vi "禹山叶绿素a校准.vi"() -> ()   [LabVIEW 2016, in "斯坦道多参数.lvlib"]
uses:
  <vilib>/Utility/miscctls.llb/LVPointTypeDef.ctl
  <vilib>/Analysis/NI_AALBase.lvlib
  <vilib>/Analysis/NI_AALPro.lvlib
  <vilib>/Utility/config.llb/NI_LVConfig.lvlib
panel:
  out "第二点校准值":dbl
  out "第一点校准值":dbl
  out "最小值":sgl format="%.2g"
  out "最大值":sgl format="%.2g"
  in  "校准停止":bool
  in  "校准模式":enum16{"两点校准", "单点校准"}(ring)
  in  "标液2":dbl
  in  "标液1":dbl
  out "波形图表":sgl(graph) caption="历史曲线"
  out "温度测量值":dbl caption="温度"
  out "变异系数":dbl format="%.6g"
  out "standard deviation":dbl caption="标准差" format="%0.2f"
  out "mean":dbl caption="均值" format="%0.2f"
  out "提示":string
  in  "校准启动":bool
  out "测试值":dbl
  out "电极斜率":dbl
  out "电极零点":dbl
  # "叶绿素a电极设定"
  # "请选择校准模式:"
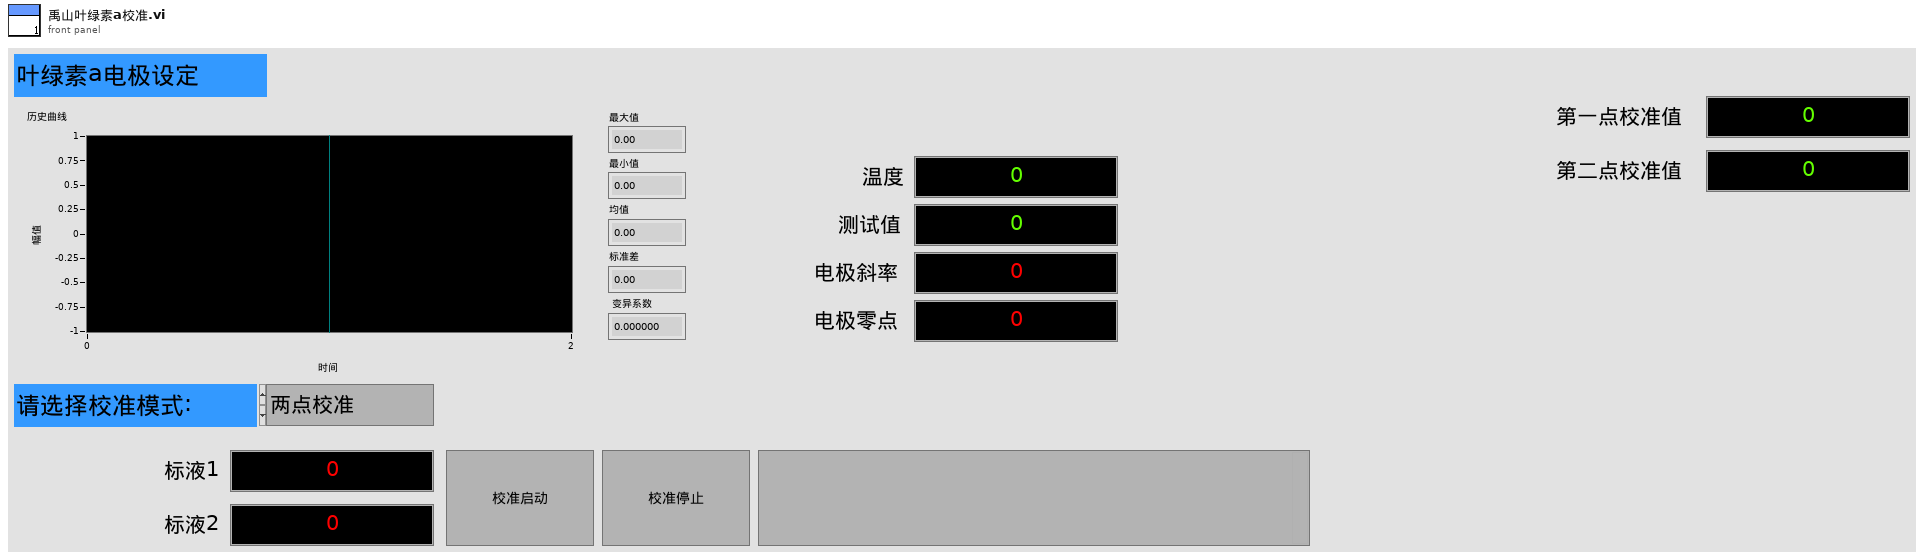
[diagram p1: front panel]
types:
  T1 = typedef "斯坦道多参数.lvlib/校准步骤.ctl" = enum16{"待机", "放置第一点标液", "第一点校准启动", "第一点校准写入", "第一点校准失败", "放置第二点标液", "第二点校准启动", "第二点校准写入", "第二点校准失败", "校准结果写入", "校准结束"}
  T2 = typedef "LVPointTypeDef.ctl" = cluster{"Horizontal":i16, "Vertical":i16}
  T3 = typedef "NI_LVConfig.lvlib/Config Data RefNum.ctl" = refnum<k1>
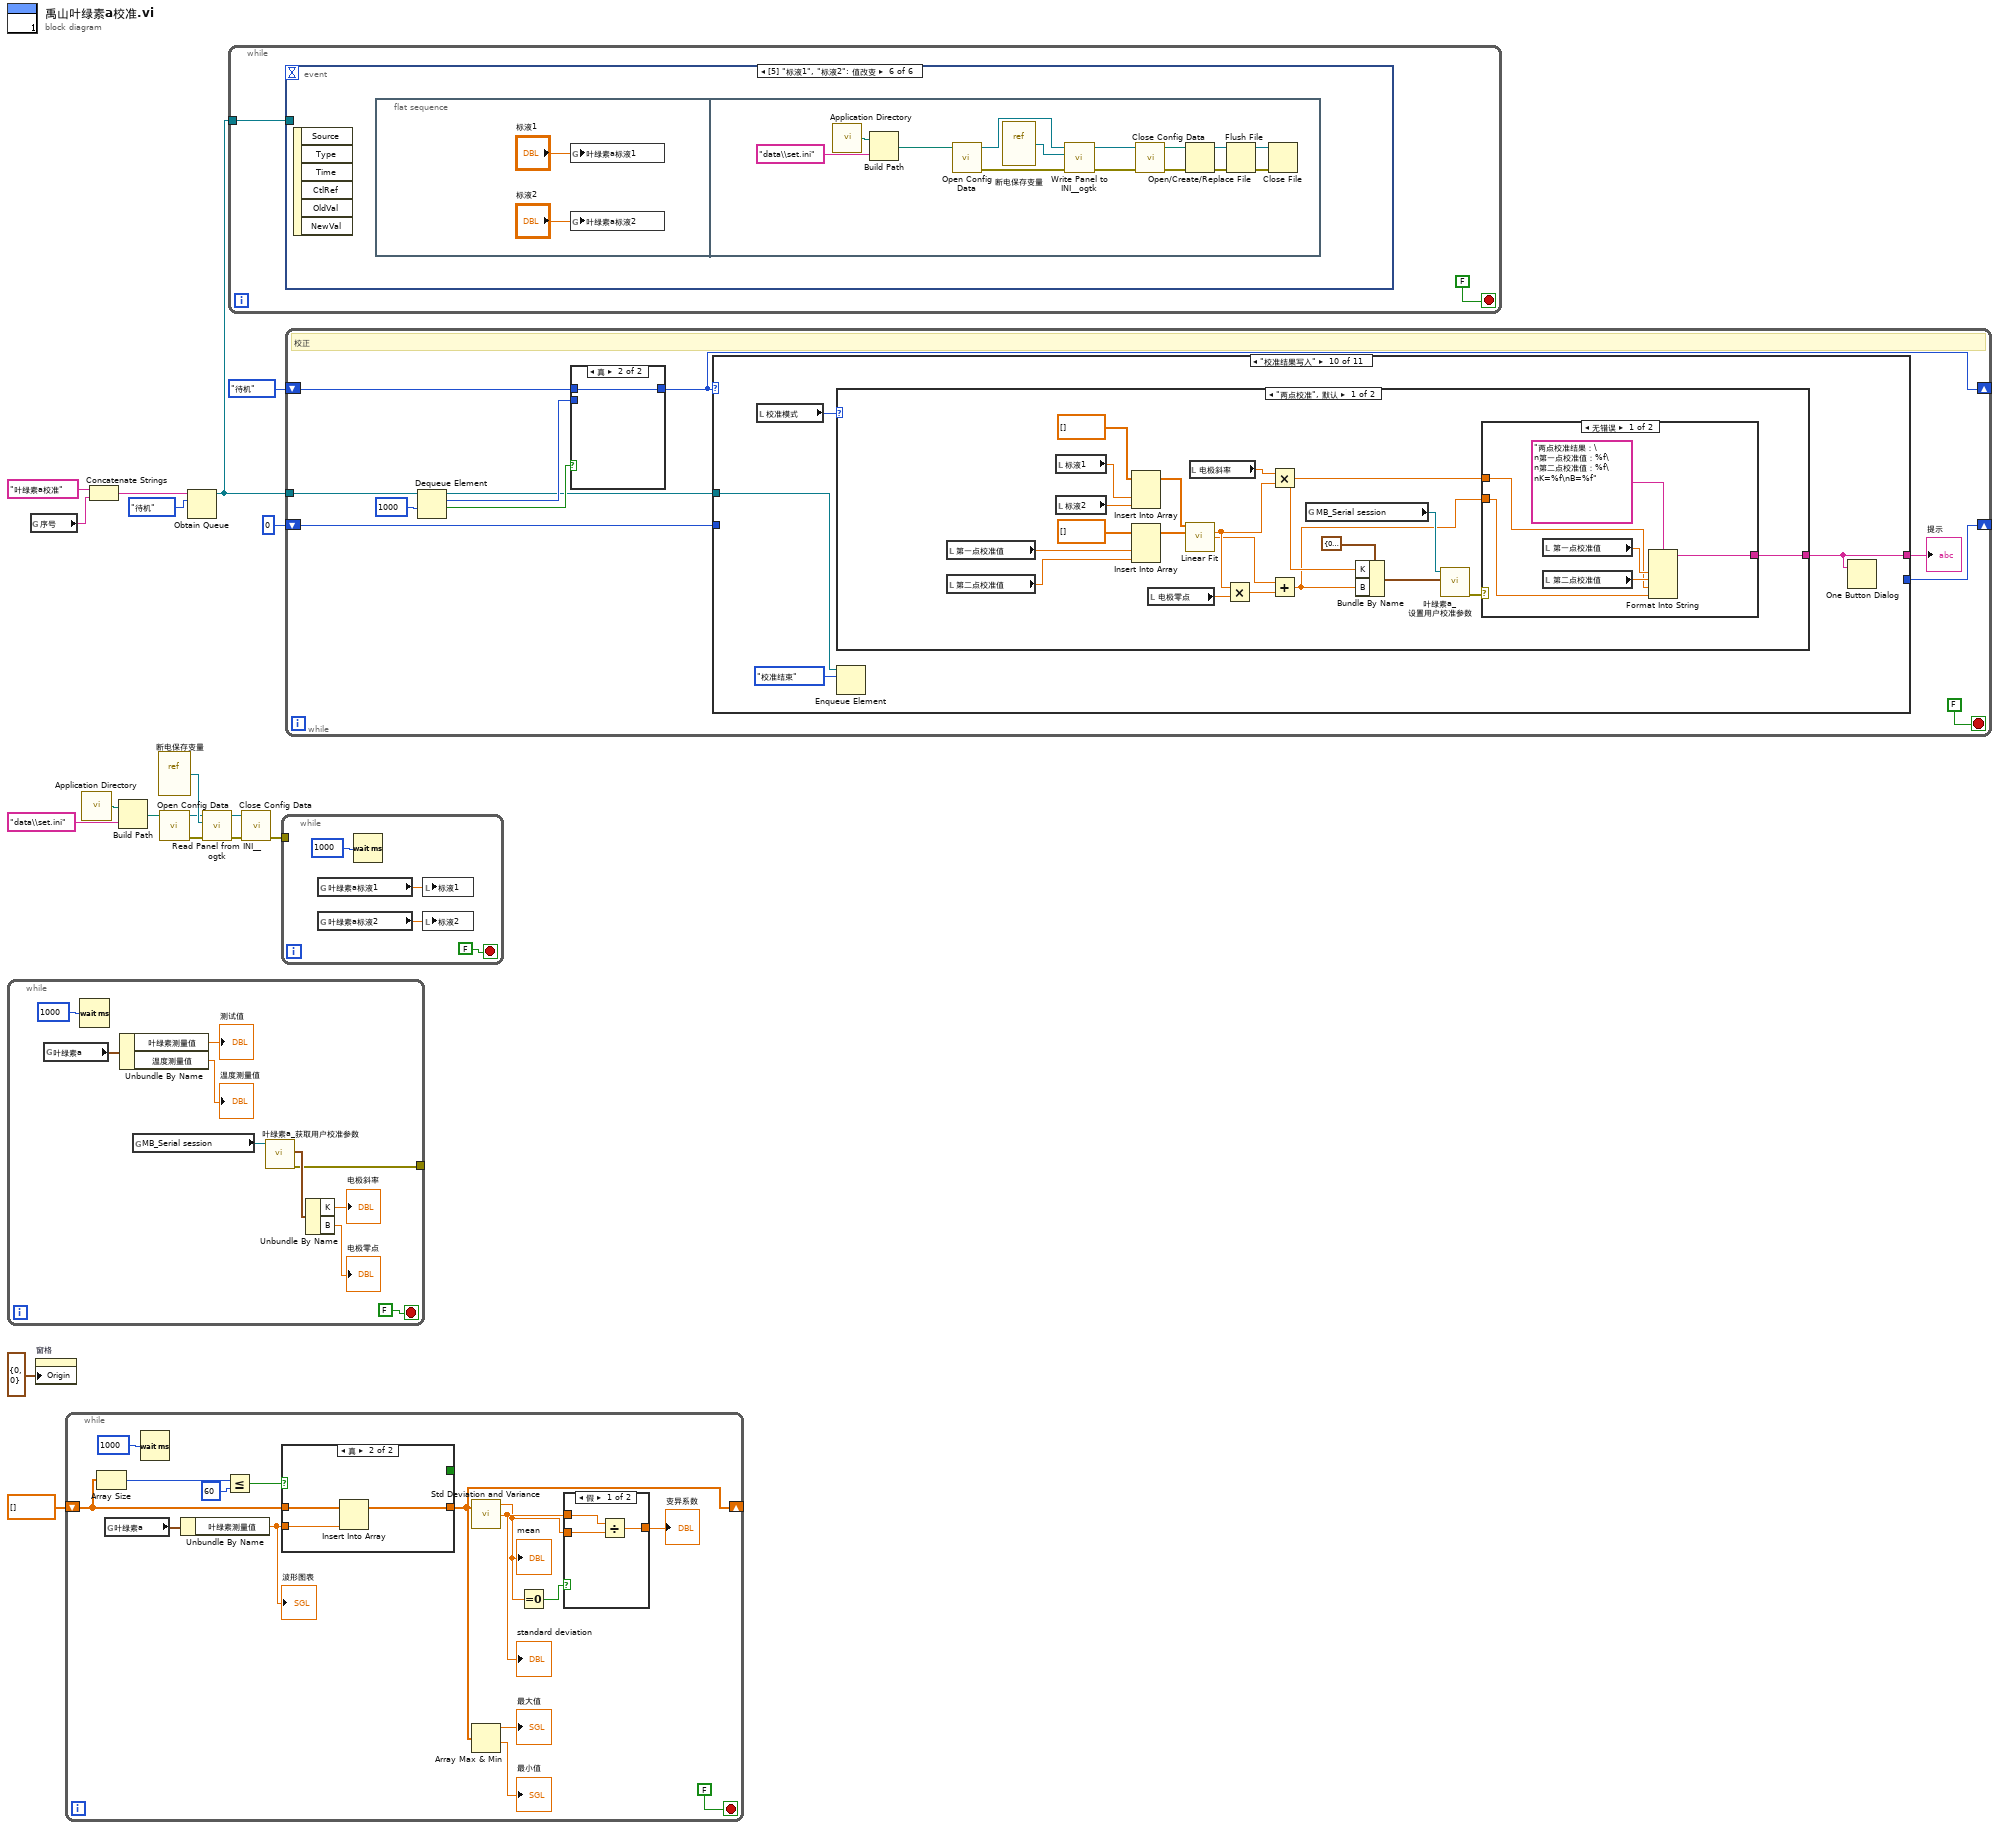
[diagram p0: block diagram]
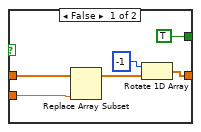
[diagram p3: hidden frame]
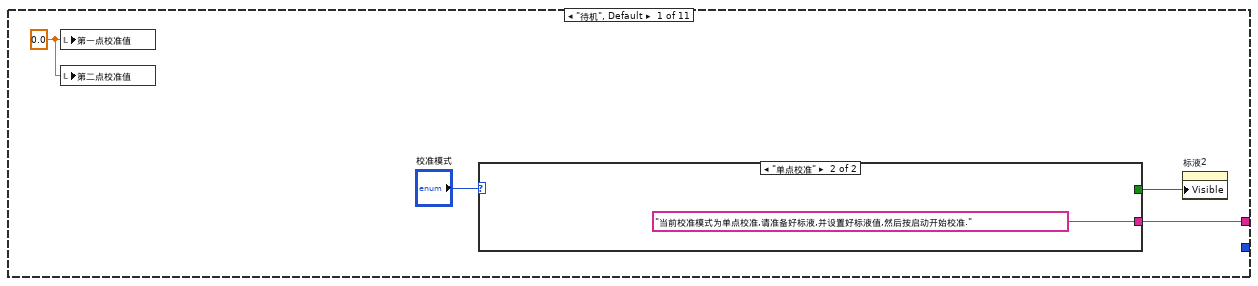
[diagram p5: hidden frame]
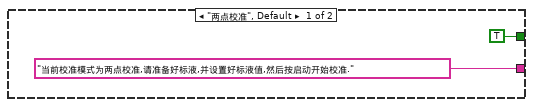
[diagram p6: hidden frame]
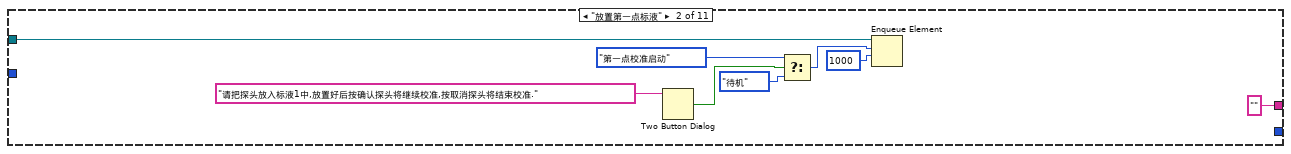
[diagram p7: hidden frame]
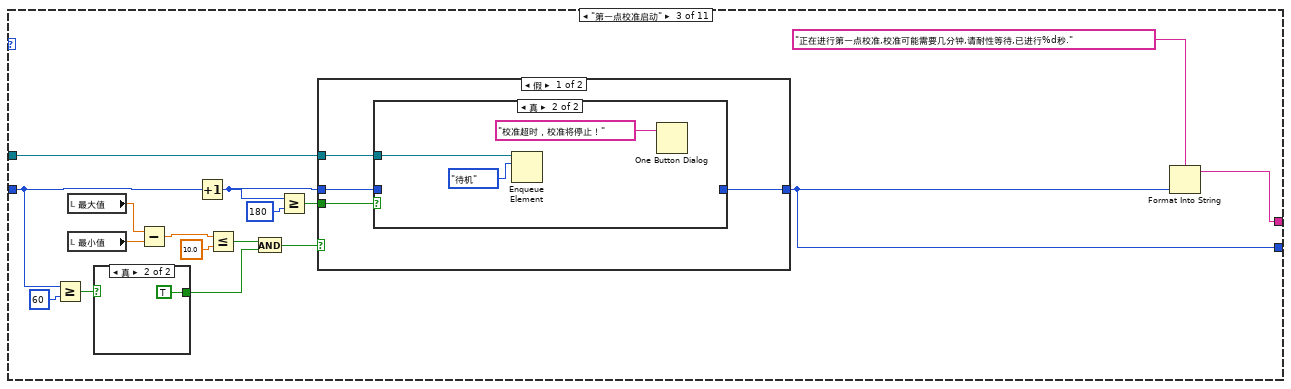
[diagram p8: hidden frame]
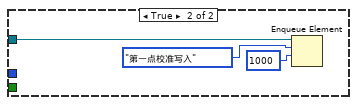
[diagram p10: hidden frame]
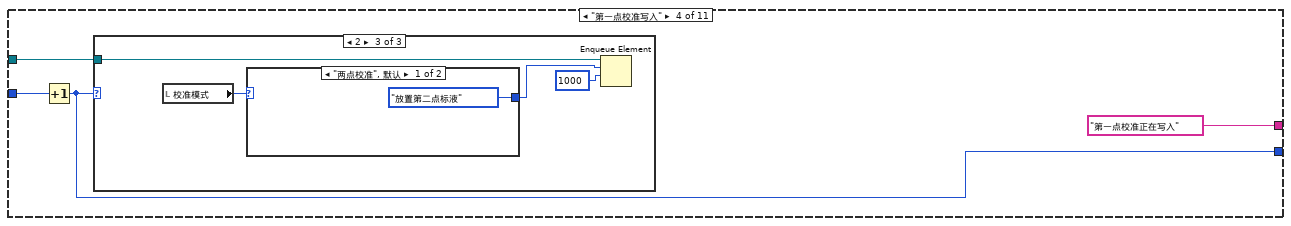
[diagram p12: hidden frame]
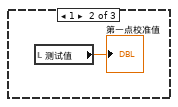
[diagram p14: hidden frame]
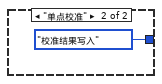
[diagram p15: hidden frame]
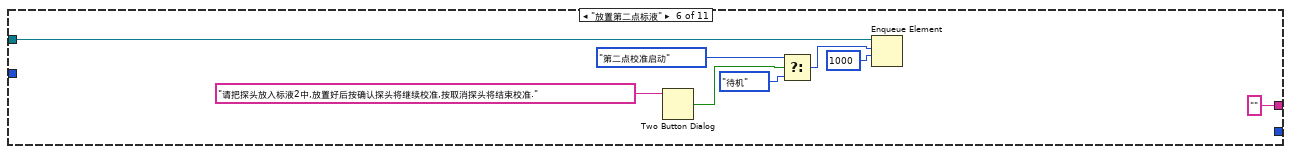
[diagram p17: hidden frame]
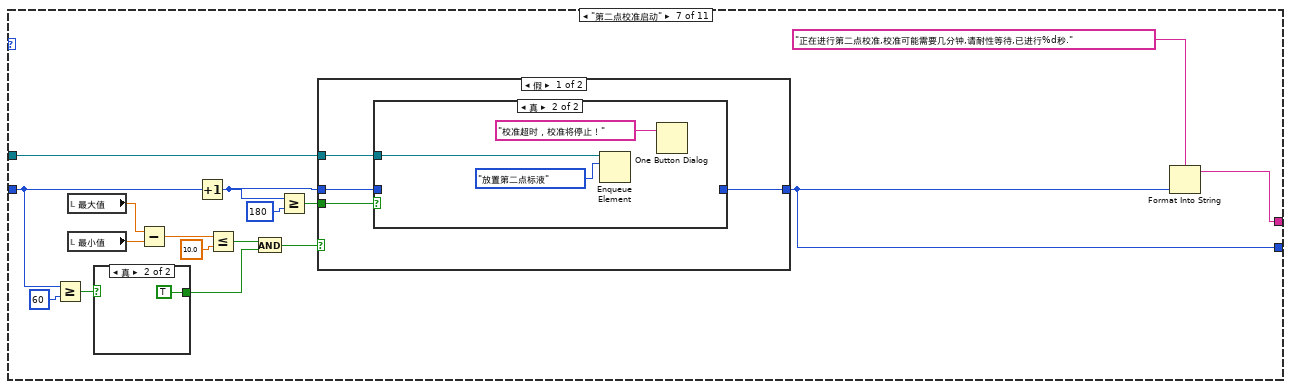
[diagram p18: hidden frame]
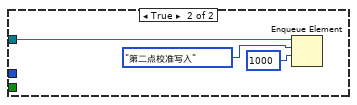
[diagram p20: hidden frame]
diagram:
  n1 = while {
    tunnel: [w23] -> _
    stop <- FALSE stop-if-true
    n2 = global read "禹山过程全局变量.vi" "叶绿素a"() -> (w20:cluster{"温度测量值":sgl, "叶绿素测量值":sgl, "错误标志":u16})
    n3 = Wait (ms)(milliseconds to wait=u32 1000 ("等待时间（毫秒）")) -> ()  [unwired: 1 out]
    n4 = Unbundle By Name(w20) -> ("叶绿素测量值"=→"测试值":sgl, "温度测量值"=→"温度测量值":sgl)
    n5 = global read "多参数全局变量.vi" "MB_Serial session"() -> (w19:refnum<class "MB_Master_Serial.lvclass">)
    n6 = call "叶绿素a_获取用户校准参数.vi"("MB_Serial session in"=w19) -> ("error out"=w23:errorcluster, "输出值"=w26:cluster{"K":sgl, "B":sgl})  [unwired: 8 in, 1 out]
    n7 = Unbundle By Name(w26) -> ("K"=→"电极斜率":sgl, "B"=→"电极零点":sgl)
  }
  n8 = global read "多参数全局变量.vi" "序号"() -> (w1:string)
  n9 = property on="窗格" class="Pane"("Origin"=T2 {"Horizontal"=0, "Vertical"=0} ("原点")) -> ()  [unwired: 2 in, 2 out]
  n10 = while {
    shift-right: [w31] -> _
    shift-left: sgl[] [] -> [w39]
    stop <- FALSE stop-if-true
    n11 = Array Size(array=w39) -> (size(s)=w41:i32)
    n12 = global read "禹山过程全局变量.vi" "叶绿素a"() -> (w33:cluster{"温度测量值":sgl, "叶绿素测量值":sgl, "错误标志":u16})
    n13 = Wait (ms)(milliseconds to wait=u32 1000 ("等待时间（毫秒）")) -> ()  [unwired: 1 out]
    n14 = Unbundle By Name(w33) -> ("叶绿素测量值"=w32:sgl)
    "波形图表" <- w32
    n15 = Less Or Equal?(x=w41, y=60) -> (x <= y?=w40:bool)
    n16 = case shown="真" w40 {
      tunnel: w39 -> [w52 w55]
      tunnel: w32 -> [w50 w54]
      tunnel: [w48 w53] -> w31
      tunnel: [TRUE _] -> _
      frame False {
        n17 = Replace Array Subset(array=w52, new element=w50) -> (w51:sgl[])  [unwired: 1 in]
        n18 = Rotate 1D Array(1:w51, 2:-1 ("n")) -> (0:w48:sgl[])
      }
      frame True {
        n19 = Insert Into Array(array=w55, new element=w54) -> (w53:sgl[])  [unwired: 1 in]
      }
    }
    n20 = call <vilib>:"Std Deviation and Variance.vi"("X"=w31) -> ("mean"=w34:dbl, "standard deviation"=w35:dbl)  [unwired: 1 in, 1 out]
    "standard deviation" <- w35
    "mean" <- w34
    n21 = Array Max & Min(array=w31) -> (max value=→"最大值":sgl, min value=→"最小值":sgl)  [unwired: 2 out]
    n22 = Equal To 0?(x=w34) -> (x = 0?=w38:bool)
    n23 = case shown="假" w38 {
      tunnel: w35 -> [w46 _]
      tunnel: [w45 _] -> w37
      tunnel: w34 -> [w44 _]
      frame False {
        n24 = Divide(x=w46, y=w44) -> (x/y=w45:dbl)
      }
      frame True {
      }
    }
    "变异系数" <- w37
  }
  n25 = call <vilib>:"Application Directory.vi"() -> ("Application Directory"=w8:path)
  n26 = Concatenate Strings("叶绿素a校准" ("名称（未命名）"), w1) -> (w2:string)
  n27 = Build Path(base path=w8, name or relative path="data\\set.ini" ("名称或相对路径")) -> (appended path=w9:path)
  n28 = vi-ref "断电保存变量.vi"() -> (w11:refnum<vi>)
  n29 = call <vilib>:"Open Config Data.vi"("configuration file path"=w9) -> ("error out"=w5:errorcluster, "refnum"=w4:T3)  [unwired: 8 in, 1 out]
  n30 = Obtain Queue(name (unnamed)=w2, element data type=校准步骤."待机" ("枚举")) -> (queue out=w12:refnum<queue>)  [unwired: 3 in, 2 out]
  n31 = call <userlib>:"Read Panel from INI__ogtk.vi"("error in (no error)"=w5, "VI ref"=w11, "refnum"=w4) -> ("error out"=w7:errorcluster, "refnum out"=w6:T3)  [unwired: 7 in]
  n32 = while {
    tunnel: w12 -> [w56]
    stop <- FALSE stop-if-true
    n33 = event shown="[5] \"标液1\", \"标液2\": 值改变" {
      selector: _ -> [_ _ _ _ _ _]
      dyn-events: _ -> [_ _ _ _ _ _]
      timeout: _ -> [_ _ _ _ _ _]
      tunnel: w56 -> [_ w59 w63 _ _ _]
      event Timeout {
        n34 = event-data() -> ()  [unwired: 1 in, 3 out]
      }
      event "校准启动": Value Change {
        n35 = event-data() -> ()  [unwired: 1 in, 6 out]
        n36 = Enqueue Element(queue=w59, element=校准步骤."放置第一点标液" ("元素")) -> ()  [unwired: 2 in, 3 out]
      }
      event "校准停止": Value Change {
        n37 = event-data() -> ()  [unwired: 1 in, 6 out]
        n38 = Flush Queue(queue=w63) -> (queue out=w60:refnum<queue>)  [unwired: 1 in, 2 out]
        n39 = Enqueue Element(queue=w60, element=校准步骤."待机" ("元素"), timeout in ms (-1)=1000 ("超时毫秒(-1)")) -> ()  [unwired: 1 in, 3 out]
      }
      event "电极零点", "电极斜率", "标液1", "标液2": Mouse Down {
        n40 = event-data() -> ("CtlRef"=w64:refnum<vi>)  [unwired: 1 in, 7 out]
        n41 = property class="DigNum (严格)"(reference=w64) -> (reference out=w65:refnum<vi>, "Value"=w66:dbl)  [unwired: 1 in, 1 out]
        n42 = call "数字键盘.vi"("OldNumber"=w66) -> ("NewNumber"=w67:sgl)
        n43 = property class="DigNum (严格)"(reference=w65, "Val(Sgnl)"=w67) -> ()  [unwired: 1 in, 2 out]
      }
      event "电极零点", "电极斜率": Value Change {
        n44 = event-data() -> ()  [unwired: 1 in, 6 out]
        n45 = local read "电极斜率"() -> (w70:dbl)
        n46 = local read "电极零点"() -> (w69:dbl)
        n47 = global read "多参数全局变量.vi" "MB_Serial session"() -> (w68:refnum<class "MB_Master_Serial.lvclass">)
        n48 = Bundle By Name(cluster=cluster{"K":sgl, "B":sgl} {"K"=0.0, "B"=0.0} ("用户校准参数"), "K"=w70, "B"=w69) -> (w71:cluster{"K":sgl, "B":sgl})
        n49 = call "叶绿素a_设置用户校准参数.vi"("用户校准参数"=w71, "MB_Serial session in"=w68) -> ()  [unwired: 8 in, 2 out]
      }
      event "标液1", "标液2": Value Change {
        n50 = event-data() -> ()  [unwired: 1 in, 6 out]
        n51 = flat-sequence {
          frame #0 {
            n52 = global write "断电保存变量.vi" "叶绿素a标液1"("标液1") -> ()
            n53 = global write "断电保存变量.vi" "叶绿素a标液2"("标液2") -> ()
          }
          frame #1 {
            n54 = call <vilib>:"Application Directory.vi"() -> ("Application Directory"=w84:path)
            n55 = Build Path(base path=w84, name or relative path="data\\set.ini" ("名称或相对路径")) -> (appended path=w83:path)
            n56 = call <vilib>:"Open Config Data.vi"("configuration file path"=w83) -> ("error out"=w87:errorcluster, "refnum"=w88:T3)  [unwired: 8 in, 1 out]
            n57 = vi-ref "断电保存变量.vi"() -> (w81:refnum<vi>)
            n58 = call <userlib>:"Write Panel to INI__ogtk.vi"("error in (no error)"=w87, "VI ref"=w81, "refnum"=w88) -> ("error out"=w85:errorcluster, "refnum out"=w86:T3)  [unwired: 7 in]
            n59 = call <vilib>:"Close Config Data.vi"("error in (no error)"=w85, "refnum"=w86) -> ("error out"=w77:errorcluster, "file path"=w78:path)  [unwired: 8 in]
            n60 = Open/Create/Replace File(file path (use dialog)=w78, error in=w77) -> (refnum out=w79:refnum<file>, error out=w80:errorcluster)  [unwired: 4 in, 1 out]
            n61 = Flush File(refnum=w79, error in=w80) -> (refnum out=w75:refnum<file>, error out=w76:errorcluster)
            n62 = Close File(refnum=w75, error in=w76) -> ()  [unwired: 2 out]
          }
        }
      }
    }
  }
  n63 = call <vilib>:"Close Config Data.vi"("error in (no error)"=w7, "refnum"=w6) -> ("error out"=w3:errorcluster)  [unwired: 8 in, 1 out]
  n64 = while {
    tunnel: w3 -> [_]
    stop <- FALSE stop-if-true
    n65 = global read "断电保存变量.vi" "叶绿素a标液1"() -> (w90:dbl)
    n66 = global read "断电保存变量.vi" "叶绿素a标液2"() -> (w89:dbl)
    n67 = Wait (ms)(milliseconds to wait=u32 1000 ("等待时间（毫秒）")) -> ()  [unwired: 1 out]
    n68 = local write "标液1"(w90) -> ()
    n69 = local write "标液2"(w89) -> ()
  }
  n70 = while "While循环" {
    shift-right: [w94] -> _
    shift-left: 校准步骤."待机" ("枚举") -> [w95]
    shift-right: [w101] -> _
    shift-left: 0 -> [w102]
    tunnel: w12 -> [w99]
    stop <- FALSE stop-if-true
    # "校正"
    n71 = Dequeue Element(queue=w99, timeout in ms (-1)=1000 ("超时毫秒(-1)")) -> (queue out=w93:refnum<queue>, element=w96:T1, timed out?=w97:bool)  [unwired: 1 in, 1 out]
    n72 = case shown="真" w97 {
      tunnel: w96 -> [w104 _]
      tunnel: [w104 w105] -> w94
      tunnel: w95 -> [_ w105]
      frame False {
      }
      frame True {
      }
    }
    n73 = case shown="\"校准结果写入\"" w94 {
      tunnel: [w109 "" ("提示") w136 "第一点校准正在写入" ("提示") _ "" ("提示") w184 "第二点校准正在写入" ("提示") _ w209 w252] -> w100
      tunnel: w102 -> [_ _ w130 w152 _ _ w178 w200 _ _ _]
      tunnel: [_ _ w121 w151 _ _ w169 w199 _ _ _] -> w101
      tunnel: w93 -> [_ w119 w124 w150 _ w167 w172 w198 _ w208 _]
      frame "待机", Default {
        w106 = 0.0 ("第一点校准值")
        n74 = local write "第一点校准值"(w106) -> ()
        n75 = local write "第二点校准值"(w106) -> ()
        n76 = case shown="\"单点校准\"" "校准模式" {
          tunnel: ["当前校准模式为两点校准,请准备好标液,并设置好标液值,然后按启动开始校准." ("提示") "当前校准模式为单点校准,请准备好标液,并设置好标液值,然后按启动开始校准." ("提示")] -> w109
          tunnel: [TRUE ("可见") _] -> w107
          frame "两点校准", Default {
          }
          frame "单点校准" {
          }
        }
        n77 = property on="标液2" class="DigNum (严格)"("Visible"=w107) -> ()  [unwired: 2 in, 2 out]
      }
      frame "放置第一点标液" {
        n78 = Two Button Dialog(message="请把探头放入标液1中,放置好后按确认探头将继续校准,按取消探头将结束校准." ("消息")) -> (T button?=w117:bool)  [unwired: 2 in]
        n79 = Select(t=校准步骤."第一点校准启动" ("元素"), s=w117, f=校准步骤."待机" ("元素")) -> (s? t:f=w114:T1)
        n80 = Enqueue Element(queue=w119, element=w114, timeout in ms (-1)=1000 ("超时毫秒(-1)")) -> ()  [unwired: 1 in, 3 out]
      }
      frame "第一点校准启动" {
        n81 = Greater Or Equal?(x=w130, y=60) -> (x >= y?=w131:bool)
        n82 = local read "最大值"() -> (w127:sgl)
        n83 = local read "最小值"() -> (w128:sgl)
        n84 = case shown="真" w131 {
          tunnel: [_ TRUE] -> w129
          frame False {
          }
          frame True {
          }
        }
        n85 = Subtract(x=w127, y=w128) -> (x-y=w126:sgl)
        n86 = Increment(x=w130) -> (x+1=w122:i32)
        n87 = Less Or Equal?(x=w126, y=10.0) -> (x <= y?=w134:bool)
        n88 = And(x=w134, y=w129) -> (x .and. y?=w125:bool)
        n89 = Greater Or Equal?(x=w122, y=180) -> (x >= y?=w123:bool)
        n90 = case shown="假" w125 {
          tunnel: w124 -> [w140 w148]
          tunnel: w123 -> [w141 _]
          tunnel: w122 -> [w139 _]
          tunnel: [w138 _] -> w121
          frame False {
            n91 = case shown="真" w141 {
              tunnel: w140 -> [_ w145]
              tunnel: w139 -> [w142 _]
              tunnel: [w142 _] -> w138
              frame False {
              }
              frame True {
                n92 = Enqueue Element(queue=w145, element=校准步骤."待机" ("元素")) -> ()  [unwired: 2 in, 3 out]
                n93 = One Button Dialog(message="校准超时，校准将停止！" ("消息")) -> ()  [unwired: 1 in, 1 out]
              }
            }
          }
          frame True {
            n94 = Enqueue Element(queue=w148, element=校准步骤."第一点校准写入" ("元素"), timeout in ms (-1)=1000 ("超时毫秒(-1)")) -> ()  [unwired: 1 in, 3 out]
          }
        }
        n95 = Format Into String(format string="正在进行第一点校准,校准可能需要几分钟,请耐性等待,已进行%d秒." ("格式字符串"), w121) -> (resulting string=w136:string)  [unwired: 2 in, 1 out]
      }
      frame "第一点校准写入" {
        n96 = Increment(x=w152) -> (x+1=w151:i32)
        n97 = case shown="2" w151 {
          tunnel: w150 -> [_ _ w158]
          frame 0, Default {
          }
          frame 1 {
            n98 = local read "测试值"() -> (→"第一点校准值":dbl)
          }
          frame 2 {
            n99 = local read "校准模式"() -> (w157:enum16{"两点校准", "单点校准"})
            n100 = case shown="\"两点校准\", 默认" w157 {
              tunnel: [校准步骤."放置第二点标液" ("元素") 校准步骤."校准结果写入" ("元素")] -> w156
              frame "两点校准", Default {
              }
              frame "单点校准" {
              }
            }
            n101 = Enqueue Element(queue=w158, element=w156, timeout in ms (-1)=1000 ("超时毫秒(-1)")) -> ()  [unwired: 1 in, 3 out]
          }
        }
      }
      frame "第一点校准失败" {
      }
      frame "放置第二点标液" {
        n102 = Two Button Dialog(message="请把探头放入标液2中,放置好后按确认探头将继续校准,按取消探头将结束校准." ("消息")) -> (T button?=w165:bool)  [unwired: 2 in]
        n103 = Select(t=校准步骤."第二点校准启动" ("元素"), s=w165, f=校准步骤."待机" ("元素")) -> (s? t:f=w162:T1)
        n104 = Enqueue Element(queue=w167, element=w162, timeout in ms (-1)=1000 ("超时毫秒(-1)")) -> ()  [unwired: 1 in, 3 out]
      }
      frame "第二点校准启动" {
        n105 = Greater Or Equal?(x=w178, y=60) -> (x >= y?=w179:bool)
        n106 = local read "最大值"() -> (w175:sgl)
        n107 = local read "最小值"() -> (w176:sgl)
        n108 = case shown="真" w179 {
          tunnel: [_ TRUE] -> w177
          frame False {
          }
          frame True {
          }
        }
        n109 = Subtract(x=w175, y=w176) -> (x-y=w174:sgl)
        n110 = Increment(x=w178) -> (x+1=w170:i32)
        n111 = Less Or Equal?(x=w174, y=10.0) -> (x <= y?=w182:bool)
        n112 = And(x=w182, y=w177) -> (x .and. y?=w173:bool)
        n113 = Greater Or Equal?(x=w170, y=180) -> (x >= y?=w171:bool)
        n114 = case shown="假" w173 {
          tunnel: w172 -> [w188 w196]
          tunnel: w171 -> [w189 _]
          tunnel: w170 -> [w187 _]
          tunnel: [w186 _] -> w169
          frame False {
            n115 = case shown="真" w189 {
              tunnel: w188 -> [_ w193]
              tunnel: w187 -> [w190 _]
              tunnel: [w190 _] -> w186
              frame False {
              }
              frame True {
                n116 = Enqueue Element(queue=w193, element=校准步骤."放置第二点标液" ("元素")) -> ()  [unwired: 2 in, 3 out]
                n117 = One Button Dialog(message="校准超时，校准将停止！" ("消息")) -> ()  [unwired: 1 in, 1 out]
              }
            }
          }
          frame True {
            n118 = Enqueue Element(queue=w196, element=校准步骤."第二点校准写入" ("元素"), timeout in ms (-1)=1000 ("超时毫秒(-1)")) -> ()  [unwired: 1 in, 3 out]
          }
        }
        n119 = Format Into String(format string="正在进行第二点校准,校准可能需要几分钟,请耐性等待,已进行%d秒." ("格式字符串"), w169) -> (resulting string=w184:string)  [unwired: 2 in, 1 out]
      }
      frame "第二点校准写入" {
        n120 = Increment(x=w200) -> (x+1=w199:i32)
        n121 = case shown="2" w199 {
          tunnel: w198 -> [_ _ w205]
          frame 0, Default {
          }
          frame 1 {
            n122 = local read "测试值"() -> (→"第二点校准值":dbl)
          }
          frame 2 {
            n123 = Enqueue Element(queue=w205, element=校准步骤."校准结果写入" ("元素"), timeout in ms (-1)=1000 ("超时毫秒(-1)")) -> ()  [unwired: 1 in, 3 out]
          }
        }
      }
      frame "第二点校准失败" {
      }
      frame "校准结果写入" {
        n124 = local read "校准模式"() -> (w206:enum16{"两点校准", "单点校准"})
        n125 = case shown="\"两点校准\", 默认" w206 {
          tunnel: [w217 w241] -> w209
          frame "两点校准", Default {
            n126 = local read "第一点校准值"() -> (w228:dbl)
            n127 = local read "第二点校准值"() -> (w227:dbl)
            n128 = local read "标液1"() -> (w225:dbl)
            n129 = local read "标液2"() -> (w224:dbl)
            n130 = Insert Into Array(array=dbl[] [] ("Weight"), new element #1=w225, new element #2=w224) -> (w223:dbl[])  [unwired: 1 in]
            n131 = Insert Into Array(array=dbl[] [] ("Weight"), new element #1=w228, new element #2=w227) -> (w222:dbl[])  [unwired: 1 in]
            n132 = local read "电极零点"() -> (w214:dbl)
            n133 = call <vilib>:"Linear Fit.vi"("Y"=w223, "X"=w222) -> ("slope"=w213:dbl, "intercept"=w211:dbl)  [unwired: 9 in, 3 out]
            n134 = local read "电极斜率"() -> (w215:dbl)
            n135 = Multiply(x=w213, y=w214) -> (x*y=w212:dbl)
            n136 = Multiply(x=w215, y=w213) -> (x*y=w216:dbl)
            n137 = Add(x=w211, y=w212) -> (x+y=w210:dbl)
            n138 = global read "多参数全局变量.vi" "MB_Serial session"() -> (w221:refnum<class "MB_Master_Serial.lvclass">)
            n139 = Bundle By Name(cluster=cluster{"K":sgl, "B":sgl} {"K"=0.0, "B"=0.0} ("用户校准参数"), "K"=w216, "B"=w210) -> (w220:cluster{"K":sgl, "B":sgl})
            n140 = call "叶绿素a_设置用户校准参数.vi"("用户校准参数"=w220, "MB_Serial session in"=w221) -> ("error out"=w218:errorcluster)  [unwired: 8 in, 1 out]
            n141 = case shown="无错误" w218 {
              tunnel: w216 -> [w232 _]
              tunnel: w210 -> [w231 _]
              tunnel: [w230 "校准失败"] -> w217
              frame No Error {
                n142 = local read "第一点校准值"() -> (w234:dbl)
                n143 = local read "第二点校准值"() -> (w235:dbl)
                n144 = Format Into String(format string="两点校准结果：\n第一点校准值：%f\n第二点校准值：%f\nK=%f\nB=%f" ("提示"), w234, w235, w232, w231) -> (resulting string=w230:string)  [unwired: 2 in, 1 out]
              }
              frame Error {
              }
            }
          }
          frame "单点校准" {
            n145 = local read "第一点校准值"() -> (w239:dbl)
            n146 = local read "电极零点"() -> (w238:dbl)
            n147 = local read "电极斜率"() -> (w240:dbl)
            n148 = Subtract(x=w238, y=w239) -> (x-y=w237:dbl)
            n149 = global read "多参数全局变量.vi" "MB_Serial session"() -> (w245:refnum<class "MB_Master_Serial.lvclass">)
            n150 = Bundle By Name(cluster=cluster{"K":sgl, "B":sgl} {"K"=0.0, "B"=0.0} ("用户校准参数"), "K"=w240, "B"=w237) -> (w244:cluster{"K":sgl, "B":sgl})
            n151 = call "叶绿素a_设置用户校准参数.vi"("用户校准参数"=w244, "MB_Serial session in"=w245) -> ("error out"=w242:errorcluster)  [unwired: 8 in, 1 out]
            n152 = case shown="错误" w242 {
              tunnel: w240 -> [w248 _]
              tunnel: w237 -> [w247 _]
              tunnel: [w246 "校准失败"] -> w241
              frame No Error {
                n153 = local read "第一点校准值"() -> (w250:dbl)
                n154 = Format Into String(format string="单点校准结果：\n第一点校准值：%f\nK=%f\nB=%f" ("提示"), w250, w248, w247) -> (resulting string=w246:string)  [unwired: 2 in, 1 out]
              }
              frame Error {
              }
            }
          }
        }
        n155 = Enqueue Element(queue=w208, element=校准步骤."校准结束" ("元素")) -> ()  [unwired: 2 in, 3 out]
        n156 = One Button Dialog(message=w209) -> ()  [unwired: 1 in, 1 out]
      }
      frame "校准结束" {
        n157 = local read "提示"() -> (w252:string)
      }
    }
    "提示" <- w100
  }
